vi "Quick NPT Config.vi"(7 "error in (no error)":errorcluster, 8 "Data Format":T1, 9 "Async_Setting":T2, 10 "Value":T3 {"Clock"."ClckEdge" items=["Rising", "Falling"]; "Clock"."ClckRate" items=["1 kS/s", "2 kS/s", "5 kS/s", "10 kS/s", "20 kS/s", "50 kS/s", "100 kS/s", "200 kS/s", "500 kS/s", "1 MS/s", "2 MS/s", "5 MS/s", "10 MS/s", "20 MS/s", "25 MS/s", "50 MS/s", "100 MS/s", "125 MS/s", "200 MS/s", "250 MS/s", "500 MS/s", "1 GS/s"]; "Input B"."Range" items=["20mv", "40mV", "50mV", "80mV", "100mV", "200mV", "400mV", "500mV", "800mV", "1 V", "2 V", "4 V", "5 V", "8 V", "10 V", "20 V"]; "Trigger"."Timeout (s)" format="%.2f"; "Input A"."Range" items=["20mv", "40mV", "50mV", "80mV", "100mV", "200mV", "400mV", "500mV", "800mV", "1 V", "2 V", "4 V", "5 V", "8 V", "10 V", "20 V"]}) -> (0 "error out":errorcluster, 1 "Device Out":i32)   [LabVIEW 2014]
uses:
  ATS-VI/ATS_ctl/ATS_Async_Ctrl.ctl
  ATS-VI/ATS_ctl/ATS_Async_Mode.ctl
  ATS-VI/ATS_ctl/ATS_ReadSamples.ctl
  ATS-VI/ATS_ctl/ATS_DMA_Channel.ctl
  ATS-VI/ATS_ctl/Coupling.ctl
  ATS-VI/ATS_ctl/Range.ctl
  ATS-VI/ATS_ctl/Impedance.ctl
  ATS-VI/ATS_ctl/Bandwidth.ctl
  ATS-VI/ATS_ctl/InputCtrl.ctl
  ATS-VI/ATS_ctl/TriggerEngine.ctl
  ATS-VI/ATS_ctl/ExtTrigRange.ctl
  ATS-VI/ATS_ctl/ExtTrigger.ctl
  ATS-VI/ATS_ctl/TriggerOperation.ctl
  ATS-VI/ATS_ctl/Trigger.ctl
  ATS-VI/ATS_ctl/ClockSource.ctl
  ATS-VI/ATS_ctl/ClockRate.ctl
  ATS-VI/ATS_ctl/ClockEdge.ctl
  ATS-VI/ATS_ctl/Clock.ctl
  ATS-VI/ATS_ctl/Record.ctl
  ATS-VI/ATS_ctl/ATS_Global.ctl
  ATS-VI/ATS_ctl/ATS_Async_Setting.ctl
  Type Defs/OCT DAQ Channel Data Type.ctl
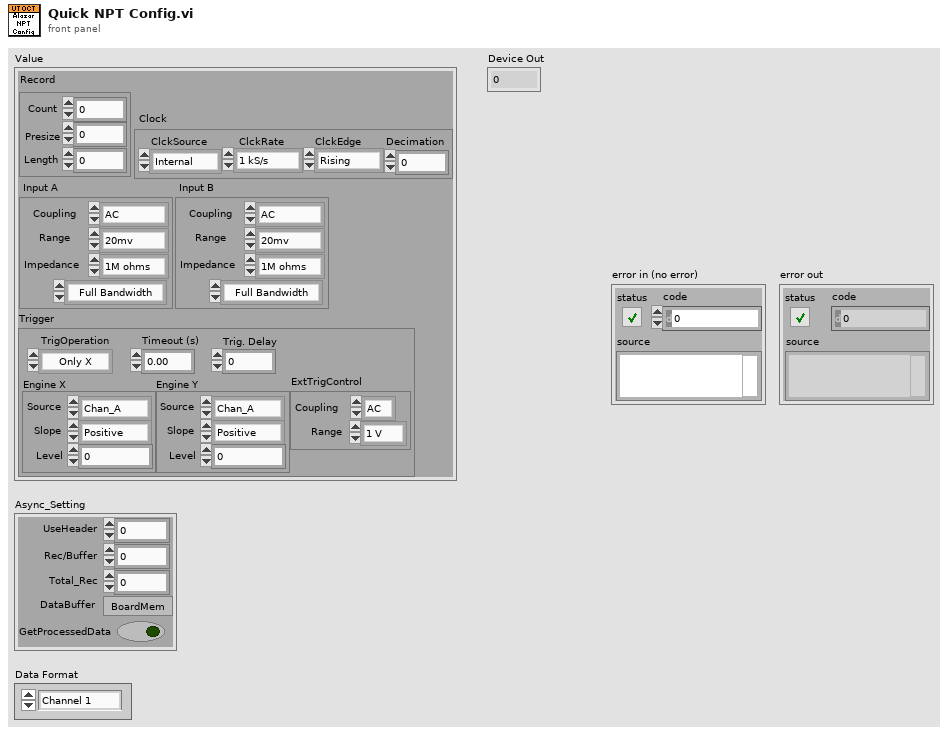
[diagram p1: front panel]
types:
  T1 = typedef "OCT DAQ Channel Data Type.ctl" = enum16{"Channel 1", "Channel 2", "Channel 1 and 2"}
  T2 = typedef "ATS_Async_Setting.ctl" = cluster{"UseHeader":u32, "Rec/Buffer":u32, "Total_Rec":u32, "DataBuffer":bool, "GetProcessedData":bool}
  T3 = typedef "ATS_Global.ctl" = cluster{"Record":T4, "Clock":T5, "Input A":T9, "Input B":T9, "Trigger":T14}
  T4 = typedef "Record.ctl" = cluster{"Count":u32, "Presize":u32, "Length":u32}
  T5 = typedef "Clock.ctl" = cluster{"ClckSource":T6, "ClckRate":T7, "ClckEdge":T8, "Decimation":u32}
  T6 = typedef "ClockSource.ctl" = enum16{"Internal", "External", "Medium Ext.", "Slow Ext.", "Ext. AC", "Ext. DC", "Ext. (PLL)"}
  T7 = typedef "ClockRate.ctl" = u32
  T8 = typedef "ClockEdge.ctl" = u16
  T9 = typedef "InputCtrl.ctl" = cluster{"Coupling":T10, "Range":T11, "Impedance":T12, "Bandwidth":T13}
  T10 = typedef "Coupling.ctl" = enum16{"AC", "DC"}
  T11 = typedef "Range.ctl" = u32
  T12 = typedef "Impedance.ctl" = enum16{"1M ohms", "50 ohms"}
  T13 = typedef "Bandwidth.ctl" = enum16{"Full Bandwidth", "Reduce Bandwidth"}
  T14 = typedef "Trigger.ctl" = cluster{"TrigOperation":T15, "Timeout (s)":dbl, "Trig. Delay":u32, "Engine X":T16, "Engine Y":T16, "ExtTrigControl":T17}
  T15 = typedef "TriggerOperation.ctl" = enum16{"Only X", "Only Y", "X or Y", "X and Y", "X xor Y", "X and not Y", "not X and Y"}
  T16 = typedef "TriggerEngine.ctl" = cluster{"Source":enum32{"Chan_A", "Chan_B", "External", "Disable"}, "Slope":enum32{"Positive", "Negative"}, "Level":u32}
  T17 = typedef "ExtTrigger.ctl" = cluster{"Coupling":T10, "Range":T18}
  T18 = typedef "ExtTrigRange.ctl" = enum16{"1 V", "5 V", "TTL"}
  T19 = typedef "ATS_ReadSamples.ctl" = cluster{"Offset":i32, "Length":u32}
  T20 = typedef "ATS_Async_Mode.ctl" = enum16{"Continuous", "Triggered", "No-Pre-Trigger", "Traditional"}
  T21 = typedef "ATS_Async_Ctrl.ctl" = enum16{"SetupDMA", "StartCapture", "Get", "Get_Stream", "Abort", "Stop"}
  T22 = typedef "ATS_DMA_Channel.ctl" = enum16{"Channel_A", "Channel_B", "A & B"}
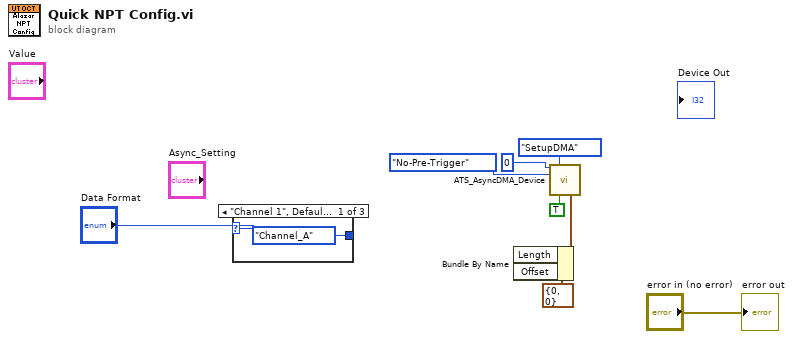
[diagram p0: block diagram]
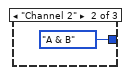
[diagram p2: hidden frame]
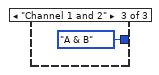
[diagram p3: hidden frame]
diagram:
  n1 = case shown="\"Channel 1\", Default" "Data Format" {
    tunnel: [ATS_DMA_Channel."Channel_A" ("Channel") ATS_DMA_Channel."A & B" ("Channel") ATS_DMA_Channel."A & B" ("Channel")] -> _
    frame "Channel 1", Default {
    }
    frame "Channel 2" {
    }
    frame "Channel 1 and 2" {
    }
  }
  n2 = Bundle By Name(cluster=T19 {"Offset"=0, "Length"=0} ("ReadSamples")) -> (w5:T19)  [unwired: 2 in]
  n3 = call "ATS_AsyncDMA_Device.vi"("DeviceIn"=0, "ATS_Async_Ctrl"=ATS_Async_Ctrl."SetupDMA" ("ATS_DMA_Ctrl"), "Async_Mode"=ATS_Async_Mode."No-Pre-Trigger", "ReadSamples"=w5, "Start Now / Wait"=TRUE) -> ()  [unwired: 6 in, 5 out]
  "error out" <- "error in (no error)"
